vi "Exp Avg Level with IC.vi"(0 "scaled signal [EU]":dbl[](array[numeric]) format="%.2f", 1 "time constant [ms]":dbl=125.0 min=0.0 format="%.2f", 2 "sampling frequency [Hz]":dbl=10000.0 format="%.2f", 3 "exponential mode":enum16{"Slow", "Fast", "Impulse", "Custom"}(ring)=enum."Fast", 4 "init/cont (init:F)":bool, 5 "initial filter state":T1 {"peak detector" format="%.2f"; "exponential averaging" format="%.2f"}) -> (6 "exp avg level [EU^2 rms]":dbl[](array[numeric]) format="%.2f", 7 "actual time constant [ms]":dbl=125.0 format="%.2f", 8 "final filter state":T1 {"peak detector" format="%.2f"; "exponential averaging" format="%.2f"})   [LabVIEW 2017]
doc: "Computes the exponential averaged level of the input signal X based on the selected exponential averaging mode and returns this level for the entire signal.\nThe initial filter state and the final filter state parameters keep track of the internal state of the filter to ensure continuous operation of the filter if continuous mode is used."
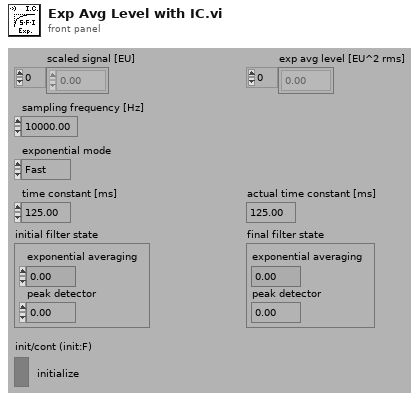
[diagram p1: front panel]
types:
  T1 = cluster{"exponential averaging":dbl, "peak detector":dbl}
  T2 = cluster{"Reverse Coefficients":dbl[], "Forward Coefficients":dbl[]}
  T3 = cluster{"final filter state":dbl, "final filter state":dbl}
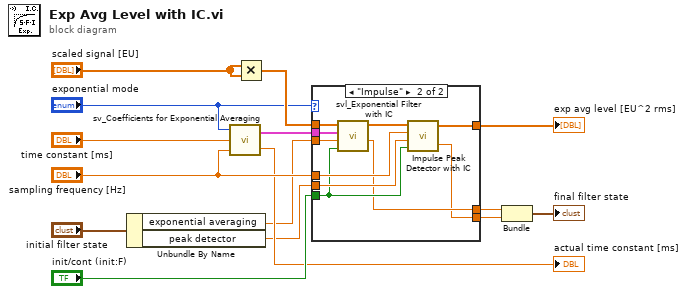
[diagram p0: block diagram]
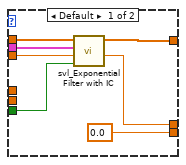
[diagram p2: hidden frame]
diagram:
  n1 = Unbundle By Name("initial filter state") -> ("exponential averaging"=w6:dbl, "peak detector"=w5:dbl)
  n2 = call <vilib>:"sv_Coefficients for Exponential Averaging.vi"("sampling frequency [Hz]"="sampling frequency [Hz]", "time constant [ms]"="time constant [ms]", "exponential mode"="exponential mode") -> ("actual time constant [ms]"=→"actual time constant [ms]":dbl, "filter coefficients"=w14:T2)
  n3 = Multiply(x="scaled signal [EU]", y="scaled signal [EU]") -> (x*y=w12:dbl[])
  n4 = case shown="\"Impulse\"" "exponential mode" {
    tunnel: w14 -> [w22 w32]
    tunnel: "init/cont (init:F)" -> [w21 w26]
    tunnel: w6 -> [w20 w31]
    tunnel: w12 -> [w19 w30]
    tunnel: "sampling frequency [Hz]" -> [_ w28]
    tunnel: w5 -> [_ w27]
    tunnel: [w18 w25] -> w4
    tunnel: [0.0 ("Final condition") w24] -> w3
    tunnel: [w16 w23] -> w1
    frame Default {
      n5 = call <vilib>:"svl_Exponential Filter with IC.vi"("init/cont (init:F)"=w21, "initial filter state"=w20, "filter coefficients"=w22, "X"=w19) -> ("final filter state"=w18:dbl, "filtered X"=w16:dbl[])  [unwired: 5 in, 1 out]
    }
    frame "Impulse" {
      n6 = call <vilib>:"svl_Exponential Filter with IC.vi"("init/cont (init:F)"=w26, "initial filter state"=w31, "filter coefficients"=w32, "X"=w30) -> ("final filter state"=w25:dbl, "filtered X"=w29:dbl[])  [unwired: 5 in, 1 out]
      n7 = call <vilib>:"Impulse Peak Detector with IC.vi"("init/cont (init:F)"=w26, "initial filter state"=w27, "sampling frequency [Hz]"=w28, "X"=w29) -> ("final filter state"=w24:dbl, "filtered X"=w23:dbl[])
    }
  }
  "exp avg level [EU^2 rms]" <- w1
  n8 = Bundle("final filter state"=w4, "final filter state"=w3) -> (→"final filter state":T3)  [unwired: 1 in]
